vi "COM_Select Modes.vi"(10 "Selection Parameters":T2, 11 "Modes IN":T1(array[cluster])) -> (3 "Modes OUT":T3[](array[typedef]))   [LabVIEW 2017, in "AppPlugins.lvlib" / "EraPlugin.lvclass"]
uses:
  EraPlugin.lvclass
  Mode/Mode Content.ctl
  COM_Select Modes Parameters.ctl
  Mode/Mode.lvclass
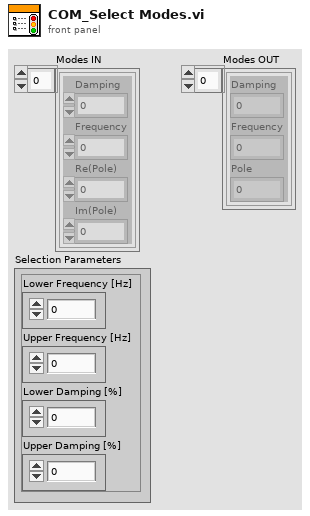
[diagram p1: front panel]
types:
  T1 = cluster{"Damping":dbl, "Frequency":dbl, "Re(Pole)":dbl, "Im(Pole)":dbl}[]
  T2 = typedef "AppPlugins.lvlib/EraPlugin.lvclass/COM_Select Modes Parameters.ctl" = cluster{"f_low":dbl, "f_up":dbl, "D_low":dbl, "D_up":dbl}
  T3 = typedef "Mode.lvclass/Mode Content.ctl" = cluster{"Damping":dbl, "Frequency":dbl, "Pole":cdb}
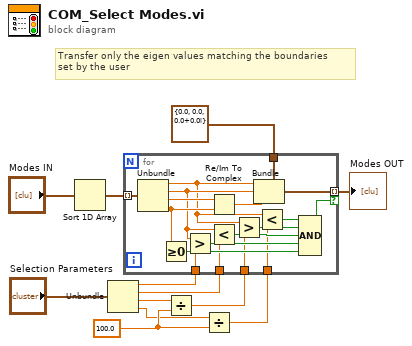
[diagram p0: block diagram]
diagram:
  w12 = 100.0 ("y")
  # "Transfer only the eigen values matching the boundaries \nset by the user"
  n1 = Sort 1D Array(array="Modes IN") -> (sorted array=w4:T1)
  n2 = Unbundle("Selection Parameters") -> ("f_low"=w5:dbl, "f_up"=w6:dbl, "D_low"=w8:dbl, "D_up"=w9:dbl)
  n3 = Divide(x=w8, y=w12) -> (x/y=w11:dbl)
  n4 = Divide(x=w9, y=w12) -> (x/y=w10:dbl)
  n5 = for {
    tunnel: w5 -> [w25]
    tunnel: w6 -> [w24]
    tunnel: w11 -> [w23]
    tunnel: w10 -> [w22]
    tunnel: w4 -> [w21] mode=indexing
    tunnel: [w13] -> w7 mode=indexing if=w20
    tunnel: T3 {"Damping"=0.0, "Frequency"=0.0, "Pole"=0.0+0.0i} ("Cluster") -> [w14]
    n6 = Unbundle(w21) -> ("Damping"=w15:dbl, "Frequency"=w16:dbl, "Re(Pole)"=w18:dbl, "Im(Pole)"=w19:dbl)
    n7 = Greater Or Equal To 0?(x=w19) -> (x >= 0?=w30:bool)
    n8 = Greater?(x=w16, y=w25) -> (0:w29:bool)
    n9 = Re/Im To Complex(1:w19, 2:w18) -> (0:w17:cdb)
    n10 = Less?(x=w16, y=w24) -> (x < y?=w28:bool)
    n11 = Greater?(x=w15, y=w23) -> (0:w27:bool)
    n12 = Bundle(cluster=w14, "Damping"=w15, "Frequency"=w16, "Pole"=w17) -> (w13:T3)
    n13 = Less?(x=w15, y=w22) -> (x < y?=w26:bool)
    n14 = Compound Arithmetic op=AND(w26, w27, w28, w29, w30) -> (w20:bool)
  }
  "Modes OUT" <- w7
